vi "Write Write Type.vi"(8 "error in":errorcluster, 10 "type":string="Not Available", 11 "Configurable Device in":refnum<class "Configurable Device.lvclass">) -> (0 "error out":errorcluster, 3 "Configurable Device out":refnum<class "Configurable Device.lvclass">)   [LabVIEW 2015, in "Configurable Device.lvclass"]
uses:
  Configurable Device.lvclass
  Configurable Device.lvclass/Configurable Device.ctl
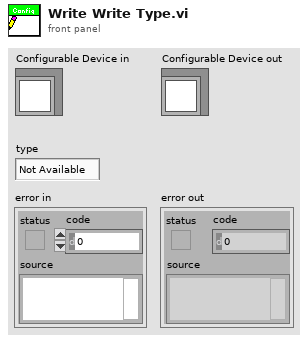
[diagram p1: front panel]
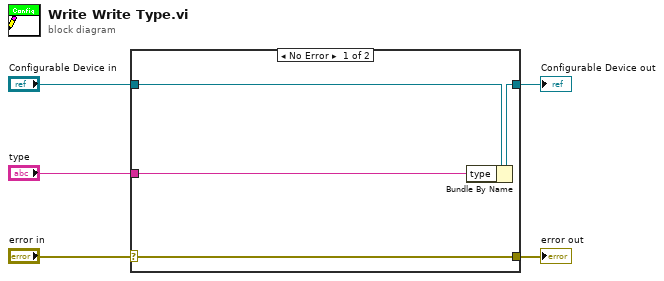
[diagram p0: block diagram]
diagram:
  n1 = case shown="No Error" "error in" {
    selector: "error in" -> [w9 w10]
    tunnel: [w9 w10] -> w4
    tunnel: [w7 w11] -> w2
    tunnel: "Configurable Device in" -> [w8 w11]
    tunnel: "type" -> [w6 _]
    frame No Error {
      n2 = Bundle By Name(cluster=w8, "type"=w6) -> (w7:refnum<class "Configurable Device.lvclass">)
    }
    frame Error {
    }
  }
  "error out" <- w4
  "Configurable Device out" <- w2
